vi "Analog Input.vi"() -> ()   [LabVIEW 2013]
doc: "Analog Input Example\n\nThis example will read voltages from an analog channel and display it on a chart. It will also display the average voltage over time. \n\nThe values for Average Bits and Samples Per Second on the front panel can be set while the VI is running.\n\nThis example works with the NI 9201 module with an Analog Breakout attached. The Analog Breakout should have 12V applied to the WAGO connector (J3). Sensors are attached to the 3x8 header using 3-pin PWM connectors. The center pin of the 3-pin connector is 5V out that can be used to power sensors. The pin closest to the PCB (Printed Circuit Board) is ground. The pin farthest from the PCB is the signal input to be read by this VI. The signal range allowed is -10 volts to +10 volts."
uses:
  <vilib>/Rock Robotics/SystemInterfaces/AI/FPGA_AIChannel.ctl
  <vilib>/Rock Robotics/SystemInterfaces/Typedef/FPGA_TypedefAnalogModule.ctl
panel:
  in  "Analog Module":T1
  in  "Samples Per Second":dbl=1000.0
  in  "Average Bits":u8=3 max=15
  in  "Channel":T2
  out "Voltage Display":cluster{"Value":dbl, "Voltage":dbl}(graph)
  out "Average Voltage":dbl
  out "Voltage":dbl
  in  "stop":bool
  # "Set these inputs before running."
  # "These can be set while running."
  # "This chart displays the voltage and average voltage over time."
  # "Wiring Diagram for Analog Breakout connected to an NI 9201"
  # "jumper to read battery or AI8"
  # "GND"
  # "SIG"
  # "5V"
  # "AI8\nAI7\nAI6\nAI5\nAI4\nAI3\nAI2\nAI1"
  # "Signal"
  # "+"
  # "12V from battery"
  # "-"
  # "Signal Ground"
  # "\"power good\" LED"
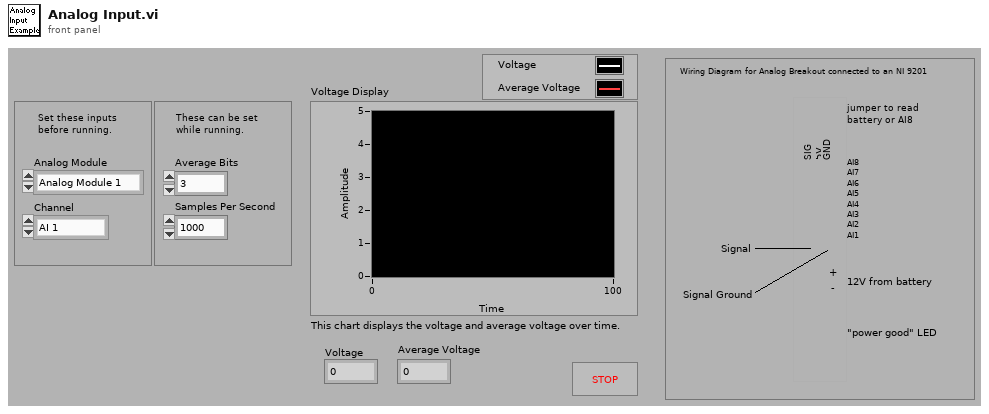
[diagram p1: front panel]
types:
  T1 = typedef "FPGA_TypedefAnalogModule.ctl" = enum16{"Analog Module 1", "Analog Module 2"}
  T2 = typedef "FPGA_AIChannel.ctl" = enum8{"AI 1", "AI 2", "AI 3", "AI 4", "AI 5", "AI 6", "AI 7", "AI 8", "Invalid"}
  T3 = typedef "WPI_AnalogChannelDevRef.ctl" = cluster{"DevStatus":errorcluster, "Analog Module":T1, "Analog Channel":T2}
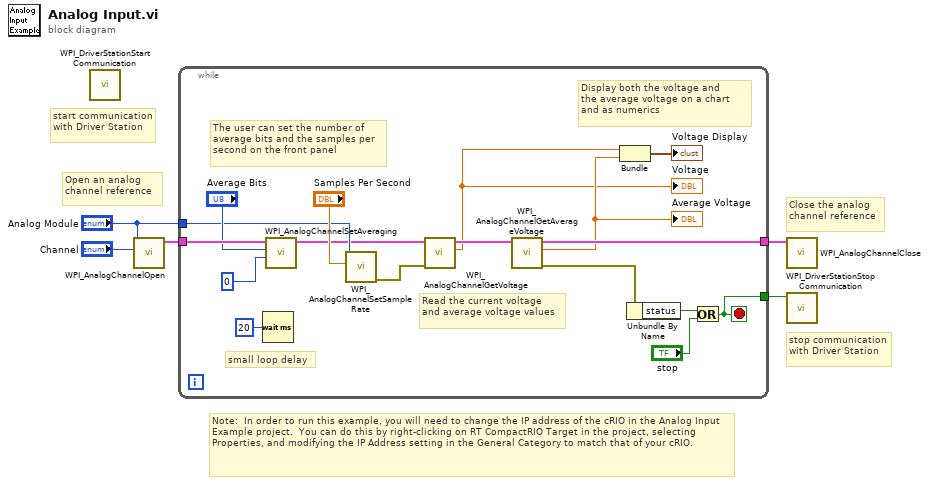
[diagram p0: block diagram]
diagram:
  # "stop communication with Driver Station"
  # "start communication with Driver Station"
  # "Close the analog\nchannel reference"
  # "Note:  In order to run this example, you will need to change the IP address of the cRIO in the Analog Input Example project.  You can do this by right-clicking on RT CompactRIO Target in the project, selecting Properties, and modifying the IP Address setting in the General Category to match that of your cRIO."
  # "Open an analog channel reference"
  n1 = call <vilib>:"WPI_DriverStationStart Communication.vi"() -> ()  [unwired: 1 in, 11 out]
  n2 = call <vilib>:"WPI_AnalogChannelOpen.vi"("Analog Channel"="Channel", "Analog Module (Module 1)"="Analog Module") -> ("AIDeviceRef"=w5:T3)  [unwired: 1 in, 8 out]
  n3 = while {
    tunnel: w5 -> [w16]
    tunnel: [w21] -> w4
    tunnel: "Analog Module" -> [w10]
    tunnel: [w6] -> w1
    stop <- w6 stop-if-true
    # "small loop delay"
    # "Read the current voltage\nand average voltage values"
    # "Display both the voltage and\nthe average voltage on a chart\nand as numerics"
    # "The user can set the number of \naverage bits and the samples per\nsecond on the front panel"
    n4 = Wait (ms)(milliseconds to wait=u32 20) -> ()  [unwired: 1 out]
    n5 = call <vilib>:"WPI_AnalogChannelSetAveraging.vi"("OversampleBits"=u8 0, "AverageBits"="Average Bits", "AIDeviceRef"=w16) -> ("AIDeviceRef"=w9:T3)  [unwired: 1 in, 7 out]
    n6 = call <vilib>:"WPI_AnalogChannelSetSampleRate.vi"("Samples Per Second"="Samples Per Second", "Analog Module (Module 1)"=w10) -> ("error out"=w7:errorcluster)  [unwired: 2 in, 7 out]
    n7 = call <vilib>:"WPI_AnalogChannelGetVoltage.vi"("error in (no error)"=w7, "AIDeviceRef"=w9) -> ("Voltage"=w19:dbl, "AIDeviceRef"=w22:T3)  [unwired: 8 out]
    "Voltage" <- w19
    n8 = call <vilib>:"WPI_AnalogChannelGetAverageVoltage.vi"("AIDeviceRef"=w22) -> ("error out"=w8:errorcluster, "Voltage"=w20:dbl, "AIDeviceRef"=w21:T3)  [unwired: 1 in, 7 out]
    "Average Voltage" <- w20
    n9 = Bundle("Voltage"=w19, "Voltage"=w20) -> (→"Voltage Display":cluster{"Voltage":dbl, "Voltage":dbl})  [unwired: 1 out]
    n10 = Unbundle By Name(w8) -> ("status"=w14:bool)
    n11 = Or(x=w14, y="stop") -> (x .or. y?=w6:bool)
  }
  n12 = call <vilib>:"WPI_AnalogChannelClose.vi"("AIDeviceRef"=w4) -> ()  [unwired: 1 in, 10 out]
  n13 = call <vilib>:"WPI_DriverStationStop Communication.vi"("StopCommunication"=w1) -> ()  [unwired: 1 in, 10 out]
